vi "connect.vi"(0 "reference":refnum<class "Graph.lvclass">, 1 "egde":refnum<class "AbstractEdge.lvclass">, 2 "p1":T1 {"y" format="%.2f"; "x" format="%.2f"}, 3 "p2":T1 {"y" format="%.2f"; "x" format="%.2f"}, 5 "error in (no error)":errorcluster) -> (14 "reference out":refnum<class "Graph.lvclass">, 15 "connected":bool, 19 "error out":errorcluster)   [LabVIEW 2014, in "Graph.lvclass"]
doc: "Adds an edge to the graph that joins the nodes containing\n the given points. If the points aren't both inside nodes,\n then no edge is added.\n @param e the edge to add\n @param p1 a point in the starting node\n @param p2 a point in the ending node\n */\n public boolean connect(Edge e, Point2D p1, Point2D p2)"
uses:
  <resource>/Framework/Providers/Open_GDS/UML/Graph_class/Graph.lvclass
  <resource>/Framework/Providers/Open_GDS/UML/AbstractEdge_class/AbstractEdge.lvclass
  <resource>/Framework/Providers/Open_GDS/UML/General/Point/Point Point2D.ctl
  <resource>/Framework/Providers/Open_GDS/UML/AbstractNode_class/AbstractNode.lvclass
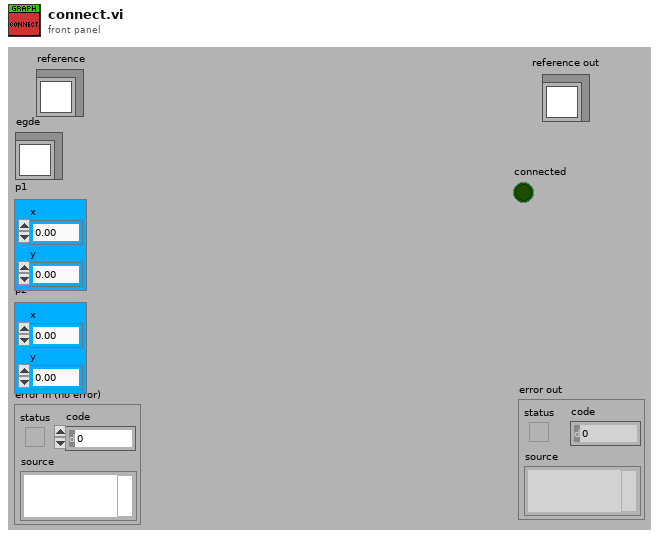
[diagram p1: front panel]
types:
  T1 = typedef "Point Point2D.ctl" = cluster{"x":dbl, "y":dbl}
  T2 = typedef "Graph.lvclass/ObjectAttributes.ctl" = cluster{"nodes":refnum<class "AbstractNode.lvclass">[], "edges":refnum<class "AbstractEdge.lvclass">[], "nodesToBeRemoved":refnum<class "AbstractNode.lvclass">[], "edgesToBeRemoved":refnum<class "AbstractEdge.lvclass">[], "needsLayout":bool, "LayoutNodes":refnum<class "AbstractNode.lvclass">[]}
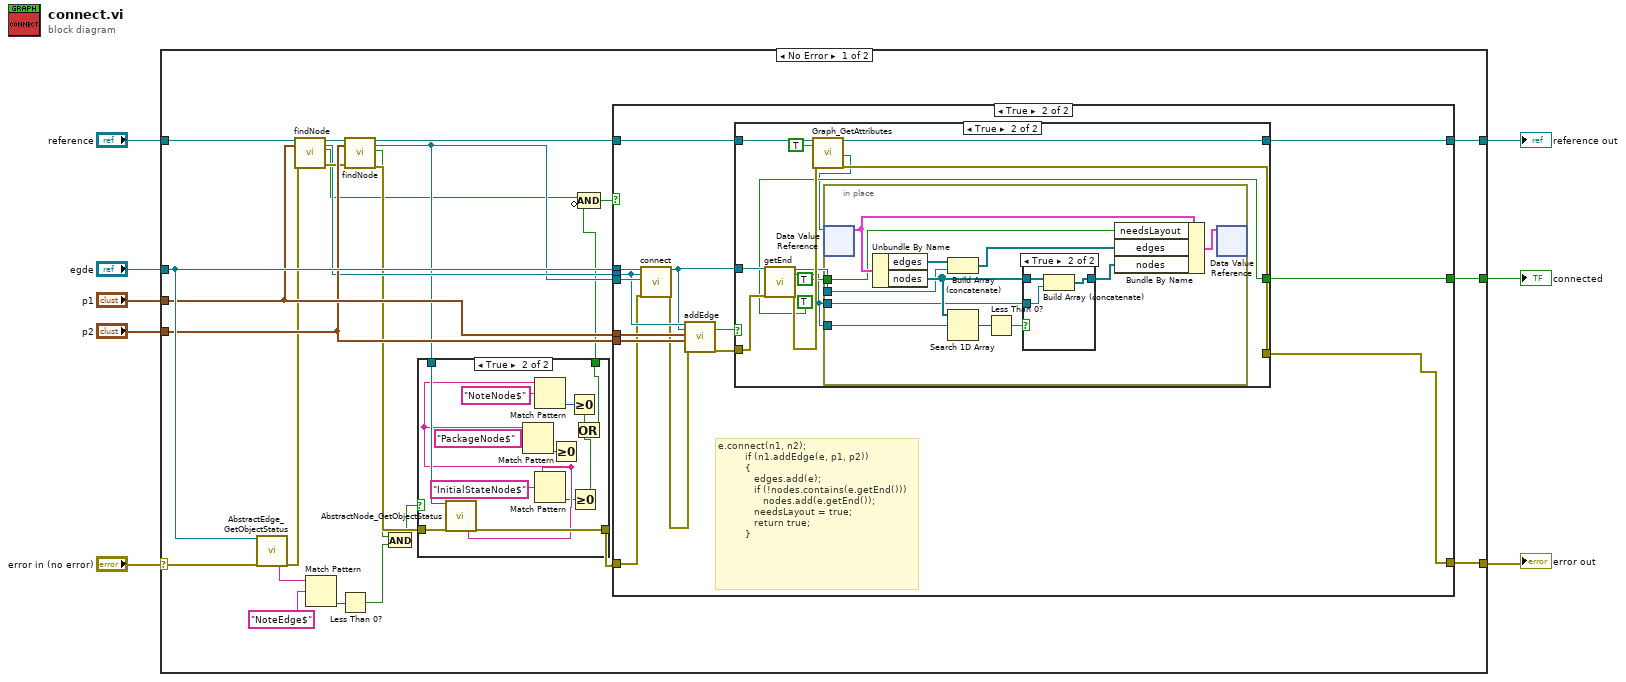
[diagram p0: block diagram]
diagram:
  n1 = case shown="No Error" "error in (no error)" {
    selector: "error in (no error)" -> [w30 w94]
    tunnel: "reference" -> [w33 w95]
    tunnel: [w32 w94] -> w7
    tunnel: [w31 w95] -> w6
    tunnel: "egde" -> [w29 _]
    tunnel: "p1" -> [w28 _]
    tunnel: "p2" -> [w27 _]
    tunnel: [w26 _] -> w1
    frame No Error {
      n2 = call <resource>:"AbstractEdge_GetObjectStatus.vi"("reference in"=w29, "error in (no error)"=w30) -> ("Class name"=w9:string, "error out"=w15:errorcluster)  [unwired: 16 out]
      n3 = call-dynamic "findNode.vi"("reference"=w33, "point2D"=w28, "error in (no error)"=w15) -> ("reference out"=w24:refnum<class "Graph.lvclass">, "node"=w22:refnum<class "AbstractNode.lvclass">, "found"=w18:bool, "error out"=w25:errorcluster)  [unwired: 13 in]
      n4 = Match Pattern(string=w9, regular expression="NoteEdge$") -> (offset past match=w11:i32)  [unwired: 4 out]
      n5 = Less Than 0?(x=w11) -> (x < 0?=w10:bool)
      n6 = call-dynamic "findNode.vi"("reference"=w24, "point2D"=w27, "error in (no error)"=w25) -> ("reference out"=w23:refnum<class "Graph.lvclass">, "node"=w19:refnum<class "AbstractNode.lvclass">, "found"=w13:bool, "error out"=w21:errorcluster)  [unwired: 13 in]
      n7 = And(x=w13, y=w10) -> (x .and. y?=w12:bool)
      n8 = case shown="True" w12 {
        tunnel: w21 -> [w34 w47]
        tunnel: [w34 w46] -> w20
        tunnel: w19 -> [_ w45]
        tunnel: [_ w35] -> w16
        frame False {
        }
        frame True {
          n9 = call <resource>:"AbstractNode_GetObjectStatus.vi"("reference in"=w45, "error in (no error)"=w47) -> ("Class name"=w40:string, "error out"=w46:errorcluster)  [unwired: 16 out]
          n10 = Match Pattern(string=w40, regular expression="PackageNode$") -> (offset past match=w42:i32)  [unwired: 4 out]
          n11 = Match Pattern(string=w40, regular expression="NoteNode$") -> (offset past match=w43:i32)  [unwired: 4 out]
          n12 = Match Pattern(string=w40, regular expression="InitialStateNode$") -> (offset past match=w38:i32)  [unwired: 4 out]
          n13 = Greater Or Equal To 0?(x=w42) -> ()  [unwired: 1 out]
          n14 = Greater Or Equal To 0?(x=w43) -> (x >= 0?=w36:bool)
          n15 = Greater Or Equal To 0?(x=w38) -> (x >= 0?=w37:bool)
          n16 = Or(x=w36, y=w37) -> (x .or. y?=w35:bool)
        }
      }
      n17 = Compound Arithmetic op=AND(w18, invert w16) -> (w17:bool)
      n18 = case shown="True" w17 {
        tunnel: [w48 w63] -> w32
        tunnel: [w49 w62] -> w31
        tunnel: w20 -> [w48 w53]
        tunnel: w23 -> [w49 w61]
        tunnel: w29 -> [_ w60]
        tunnel: w22 -> [_ w58]
        tunnel: w19 -> [_ w59]
        tunnel: w28 -> [_ w57]
        tunnel: w27 -> [_ w56]
        tunnel: [_ w50] -> w26
        frame False {
        }
        frame True {
          # "e.connect(n1, n2);\n         if (n1.addEdge(e, p1, p2))\n         {\n            edges.add(e);\n            if (!nodes.contains(e.getEnd()))\n               nodes.add(e.getEnd());\n            needsLayout = true;\n            return true;\n         }"
          n19 = call-dynamic "connect.vi"("reference"=w60, "startNode"=w58, "endNode"=w59, "error in (no error)"=w53) -> ("reference out"=w54:refnum<class "AbstractEdge.lvclass">, "error out"=w52:errorcluster)  [unwired: 14 in]
          n20 = call-dynamic "addEdge.vi"("reference"=w58, "egde"=w54, "p1"=w57, "p2"=w56, "error in (no error)"=w52) -> ("edgeHasEndNode"=w55:bool, "error out"=w51:errorcluster)  [unwired: 12 in, 1 out]
          n21 = case shown="True" w55 {
            tunnel: [w64 w77] -> w63
            tunnel: [w65 w76] -> w62
            tunnel: w61 -> [w65 w75]
            tunnel: w51 -> [w64 w73]
            tunnel: w54 -> [_ w74]
            tunnel: [_ TRUE ("needsLayout")] -> w50
            frame False {
            }
            frame True {
              n22 = call-dynamic "getEnd.vi"("reference"=w74, "error in (no error)"=w73) -> ("reference out"=w67:refnum<class "AbstractEdge.lvclass">, "endNode"=w66:refnum<class "AbstractNode.lvclass">, "error out"=w72:errorcluster)  [unwired: 14 in, 1 out]
              n23 = call <resource>:"Graph_GetAttributes.vi"("reference in"=w75, "OnlyGetDvrReference(False)"=TRUE, "error in (no error)"=w72) -> ("reference out"=w76:refnum<class "Graph.lvclass">, "DataRef"=w69:refnum<data-value>, "error out"=w77:errorcluster)  [unwired: 13 in, 1 out]
              n24 = in-place {
                in-place-border: TRUE ("needsLayout") -> [w86]
                in-place-border: w67 -> [w82]
                in-place-border: w66 -> [w80]
                in-place-border: w66 -> [w79]
                n25 = in-place-dvr #1(w69) -> (w89:T2)  [unwired: 1 out]
                n26 = Unbundle By Name(w89) -> ("edges"=w88:refnum<class "AbstractEdge.lvclass">[], "nodes"=w87:refnum<class "AbstractNode.lvclass">[])
                n27 = Build Array (concatenate)(w88, w82) -> (w85:refnum<class "AbstractEdge.lvclass">[])
                n28 = Search 1D Array(1D array=w87, element=w79) -> (index of element=w78:i32)  [unwired: 1 out]
                n29 = Less Than 0?(x=w78) -> (x < 0?=w81:bool)
                n30 = case shown="True" w81 {
                  tunnel: w87 -> [w90 w93]
                  tunnel: [w90 w92] -> w84
                  tunnel: w80 -> [_ w91]
                  frame False {
                  }
                  frame True {
                    n31 = Build Array (concatenate)(w93, w91) -> (w92:refnum<class "AbstractNode.lvclass">[])
                  }
                }
                n32 = Bundle By Name(cluster=w89, "needsLayout"=w86, "edges"=w85, "nodes"=w84) -> (w83:T2)
                n33 = in-place-dvr #1(w83) -> ()  [unwired: 2 out]
              }
            }
          }
        }
      }
    }
    frame Error {
    }
  }
  "reference out" <- w6
  "error out" <- w7
  "connected" <- w1
